vi "rad_Create AppImage ZIP File.vi"(8 "error in (no error)":errorcluster, 10 "Source directory":path, 11 "New ZIP File path":path) -> (0 "error out":errorcluster, 3 "New ZIP File path":path)   [LabVIEW 2023]
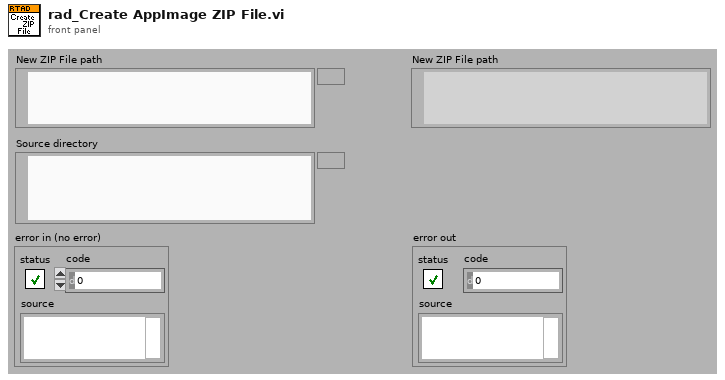
[diagram p1: front panel]
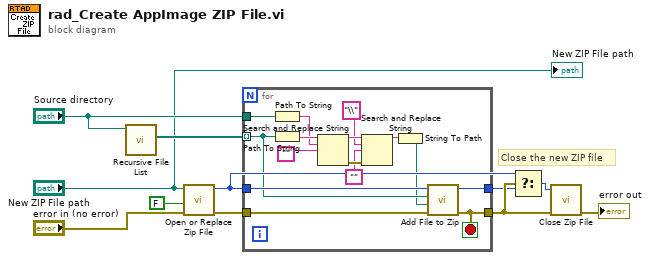
[diagram p0: block diagram]
diagram:
  # "Close the new ZIP file"
  n1 = call <vilib>:"Recursive File List.vi"("Folder Path"="Source directory") -> ("All Files in Dir"=w6:path[])  [unwired: 2 in, 8 out]
  n2 = call "Open or Replace Zip File.vi"("error in (no error)"="error in (no error)", "Replace (T) or Open?"=FALSE, "target"="New ZIP File path") -> ("error out"=w4:errorcluster, "zip file out"=w2:i64)  [unwired: 2 in, 1 out]
  n3 = for {
    tunnel: [w17] -> w10
    tunnel: [w26] -> w9
    tunnel: w6 -> [w23] mode=indexing
    tunnel: w2 -> [w25]
    tunnel: w4 -> [w24]
    tunnel: "Source directory" -> [w22]
    stop <- w17 stop-if-true
    n4 = Path To String(path=w22) -> (string=w20:string)
    n5 = Path To String(path=w23) -> (string=w21:string)
    n6 = Search and Replace String(input string=w21, search string=w20, replace string="") -> (result string=w16:string, error out=w15:errorcluster)  [unwired: 1 in, 6 out]
    n7 = Search and Replace String(input string=w16, search string="\\", replace string="", error in=w15) -> (result string=w12:string)  [unwired: 7 out]
    n8 = String To Path(string=w12) -> (path=w18:path)
    n9 = call <vilib>:"Add File to Zip.vi"("error in (no error)"=w24, "destination path in zip"=w18, "source file path"=w23, "zip file in"=w25) -> ("error out"=w17:errorcluster, "zip file out"=w26:i64)  [unwired: 6 out]
  }
  n10 = Select(t=w2, s=w10, f=w9) -> (s? t:f=w8:i64)
  n11 = call <vilib>:"Close Zip File.vi"("error in (no error)"=w10, "zip file in"=w8) -> ("error out"=→"error out":errorcluster)  [unwired: 1 in, 4 out]
  "New ZIP File path" <- "New ZIP File path"
